vi "GetSetPointCommand.vi"(11 "Set Point":dbl) -> (3 "Command":u8[](array[numeric]) format="%x")   [LabVIEW 2017]
uses:
  <instrlib>/Samwontech TEMP2xxx/Samwontech TEMP2xxx.lvlib
panel:
  out "Command":string
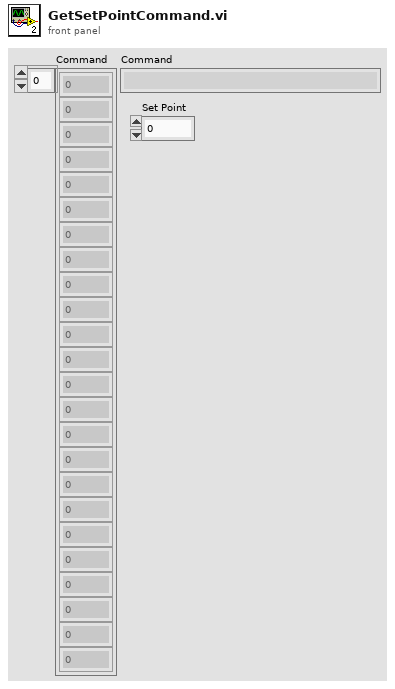
[diagram p1: front panel]
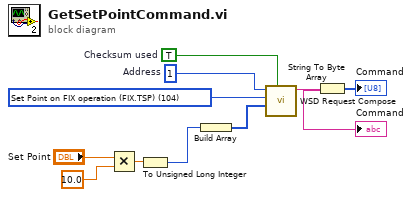
[diagram p0: block diagram]
diagram:
  w9 = u8 1  # Address
  w10 = TRUE  # Checksum used
  w8 = u32 104 items=["Current PV (NPV)"=1, "Operation Control (COM.OPMODE)"=102, "Set Point on FIX operation (FIX.TSP)"=104, "Operation Mode (OP.MODE)"=106] ("D-Registers Map")
  n1 = Multiply(x="Set Point", y=10.0) -> (x*y=w2:dbl)
  n2 = To Unsigned Long Integer(number=w2) -> (unsigned 32bit integer=w1:u32)
  n3 = Build Array(w1) -> (w7:u32[])
  n4 = call <instrlib>:"WSD Request Compose.vi"("Checksum used"=w10, "Data"=w7, "D-register number"=w8, "Address"=w9) -> ("Request"=w6:string)  [unwired: 6 in, 1 out]
  "Command" <- w6
  n5 = String To Byte Array(string=w6) -> (unsigned byte array=→"Command":u8[])
